vi "Create_File.vi"(1 "String":string) -> (0 "path":path)   [LabVIEW 2009]
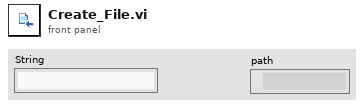
[diagram p1: front panel]
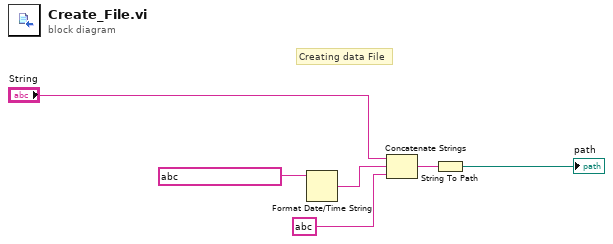
[diagram p0: block diagram]
diagram:
  # "Creating data File"
  n1 = Format Date/Time String(time format string (%c)=string ?) -> (date/time string=w6:string)  [unwired: 2 in]
  n2 = Concatenate Strings("String", w6, string ?) -> (w3:string)
  n3 = String To Path(string=w3) -> (path=→"path":path)
